vi "WD_Search_barcode.vi"(8 "error in (no error)":errorcluster, 10 "workplace_name_id":i16, 11 "DBlink":string="Driver={ODBC Driver 17 for SQL Server};Server=localhost\\SQLEXPRESS;Database=ZDX201;UID=labview;PWD=Dsa@54137926") -> (0 "error out":errorcluster, 1 "workplace_data":cluster{"條碼R":string, "條碼L":string}, 2 "找到":bool, 3 "取得ID":i16)   [LabVIEW 2019]
uses:
  <vilib>/addons/database/Connection.llb/DB Tools Open Connec (String).vi
  <vilib>/addons/database/Connection.llb/Conn Execute.vi
  <vilib>/addons/database/Recordset.llb/Rec Fetch Recordset Data (R).vi
  <vilib>/addons/database/Recordset.llb/Rec Destroy - Connection.vi
  <vilib>/addons/database/_DB Variant To Data/Database Variant To Data.xnode
  <vilib>/addons/database/NI_Database_API.lvlib
panel:
  out "size(s)":i32
  out "查詢結果":string="SELECT \n       [barcode A]\n      ,[barcode B]\n  FROM [ZDX201].[dbo].[workplace_data]\n  where [workplace_name_id]>9 and [workplace_name_id]<11 and ([barcode A] is not null or [barcode B] is not null)\n  order by [workplace_name_id]"
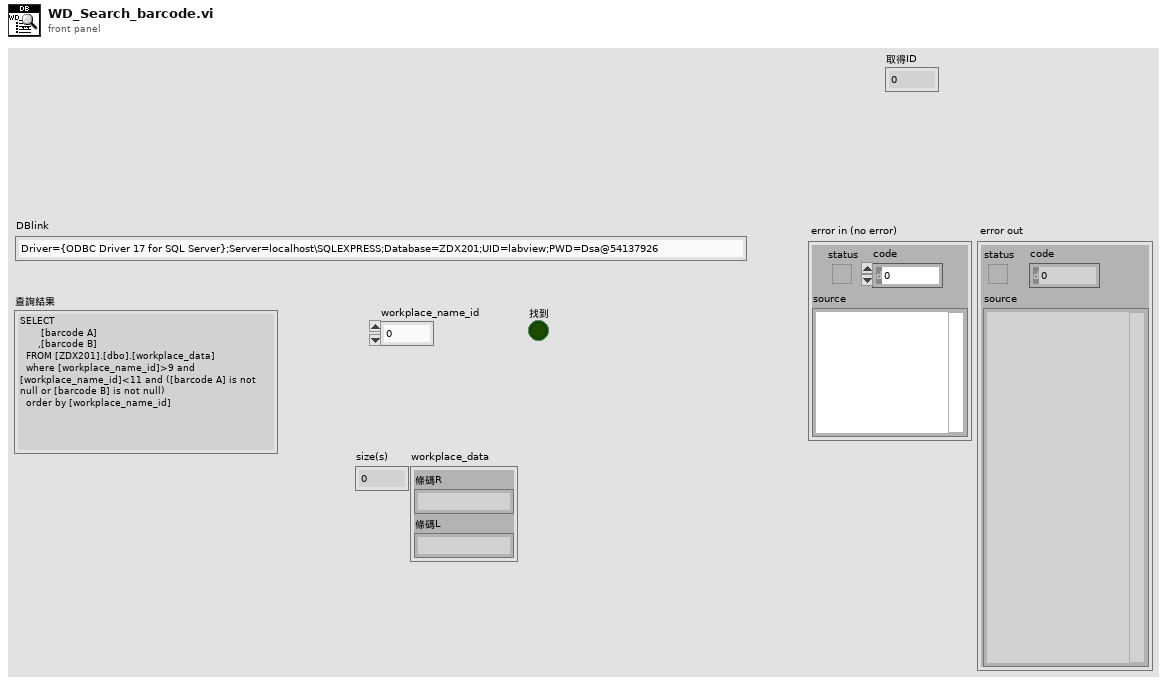
[diagram p1: front panel]
types:
  T1 = typedef "NI_Database_API.lvlib/Conn ObjectReference.ctl" = refnum<k1>
  T2 = typedef "NI_Database_API.lvlib/Rec ObjectReference.ctl" = refnum<k1>
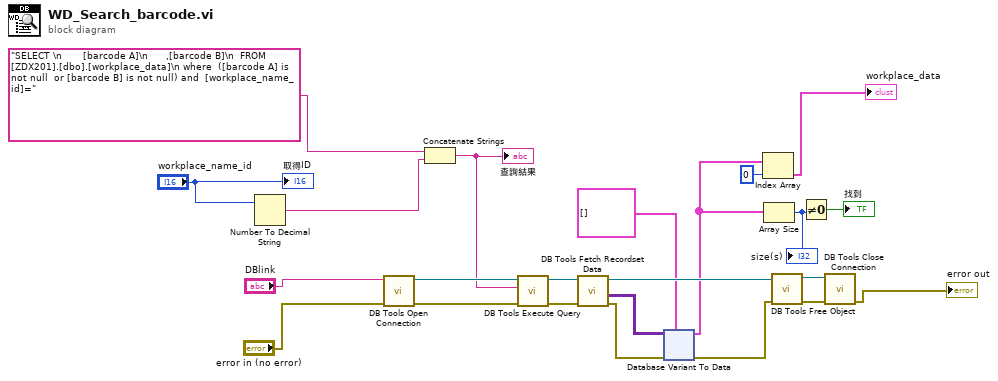
[diagram p0: block diagram]
diagram:
  n1 = Number To Decimal String(number="workplace_name_id") -> (decimal integer string=w7:string)  [unwired: 1 in]
  n2 = call-poly <vilib>:"DB Tools Open Connection.vi"("error in (no error)"="error in (no error)", "connection information"="DBlink") -> ("error out"=w23:errorcluster, "connection reference"=w22:T1)  [unwired: 6 in]
  n3 = Concatenate Strings("SELECT \n       [barcode A]\n      ,[barcode B]\n  FROM [ZDX201].[dbo].[workplace_data]\n where  ([barcode A] is not null  or [barcode B] is not null) and  [workplace_name_id]=", w7) -> (w6:string)
  "查詢結果" <- w6
  n4 = call-poly <vilib>:"DB Tools Execute Query.vi"("error in (no error)"=w23, "SQL query"=w6, "connection reference"=w22) -> ("error out"=w20:errorcluster, "recordset reference"=w21:T2)  [unwired: 5 in]
  n5 = call-poly <vilib>:"DB Tools Fetch Recordset Data.vi"("error in (no error)"=w20, "recordset reference"=w21) -> ("error out"=w15:errorcluster, "recordset data"=w14:variant[][], "recordset reference out"=w16:T2)  [unwired: 3 in]
  n6 = xnode "Database Variant To Data"("database variant"=w14, "error in (no error)"=w15, "type"=cluster{"條碼A":string, "條碼B":string}[] [] ("Workplace: assemble")) -> ("data"=w3:cluster{"條碼A":string, "條碼B":string}[], "error out"=w17:errorcluster)
  n7 = Index Array(array=w3, index=0) -> (element=→"workplace_data":cluster{"條碼A":string, "條碼B":string})
  n8 = Array Size(array=w3) -> (size(s)=w5:i32)
  "size(s)" <- w5
  n9 = call-poly <vilib>:"DB Tools Free Object.vi"("error in (no error)"=w17, "recordset reference"=w16) -> ("error out"=w18:errorcluster, "connection reference"=w19:T1)  [unwired: 8 in]
  n10 = Not Equal To 0?(x=w5) -> (x != 0?=→"找到":bool)
  n11 = call <vilib>:"DB Tools Close Connection.vi"("error in (no error)"=w18, "connection reference"=w19) -> ("error out"=→"error out":errorcluster)  [unwired: 5 in]
  "取得ID" <- "workplace_name_id"
